vi "Get Data Value.vi"(8 "error in (no error)":errorcluster, 11 "stringPayload in":refnum<class "stringPayload.lvclass">) -> (0 "error out":errorcluster, 1 "Data":string, 3 "stringPayload out":refnum<class "stringPayload.lvclass">)   [LabVIEW 2017, in "messagesPayload.lvlib" / "stringPayload.lvclass"]
uses:
  stringPayload.lvclass
  stringPayload.lvclass/stringPayload.ctl
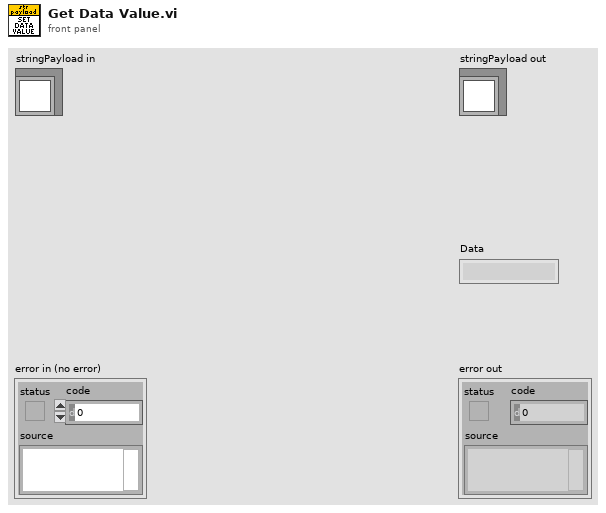
[diagram p1: front panel]
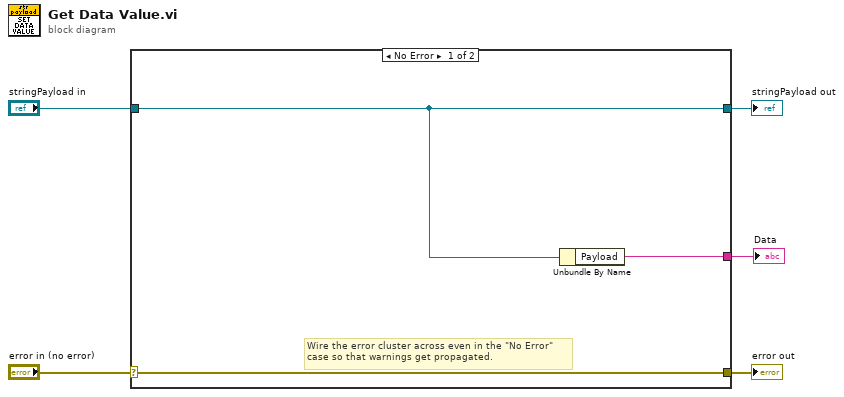
[diagram p0: block diagram]
diagram:
  n1 = case shown="No Error" "error in (no error)" {
    selector: "error in (no error)" -> [w8 w10]
    tunnel: [w8 w10] -> w4
    tunnel: [w7 w9] -> w2
    tunnel: "stringPayload in" -> [w7 w9]
    tunnel: [w6 _] -> w1
    frame No Error {
      # "Wire the error cluster across even in the \"No Error\"\ncase so that warnings get propagated."
      n2 = Unbundle By Name(w7) -> ("Payload"=w6:string)
    }
    frame Error {
    }
  }
  "error out" <- w4
  "stringPayload out" <- w2
  "Data" <- w1
